vi "Write Context.vi"(8 "error in (no error)":errorcluster, 10 "context":string, 11 "URI in":refnum<class "URI.lvclass">) -> (0 "error out":errorcluster, 3 "URI out":refnum<class "URI.lvclass">)   [LabVIEW 2013, in "openURI.lvlib" / "URI.lvclass"]
uses:
  URI.lvclass
  URI.lvclass/URI.ctl
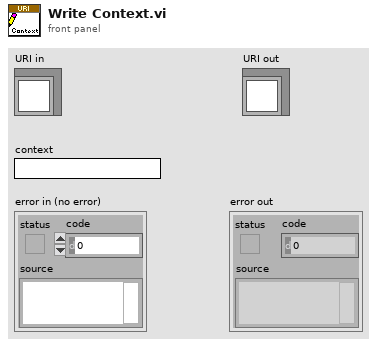
[diagram p1: front panel]
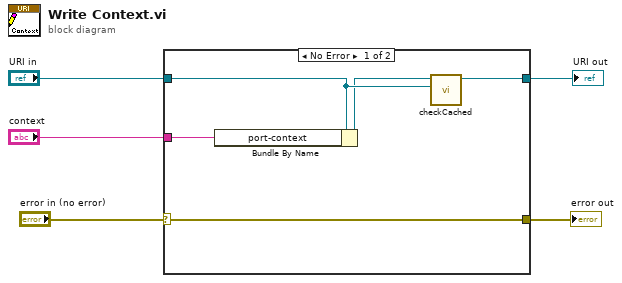
[diagram p0: block diagram]
diagram:
  n1 = case shown="No Error" "error in (no error)" {
    selector: "error in (no error)" -> [w9 w11]
    tunnel: "URI in" -> [w8 w12]
    tunnel: "context" -> [w10 _]
    tunnel: [w6 w12] -> w3
    tunnel: [w9 w11] -> w1
    frame No Error {
      n2 = Bundle By Name(cluster=w8, "port-context"=w10) -> (w7:refnum<class "URI.lvclass">)
      n3 = call "checkCached.vi"("Old"=w8, "New URI"=w7) -> ("URI"=w6:refnum<class "URI.lvclass">)  [unwired: 9 in]
    }
    frame Error {
    }
  }
  "URI out" <- w3
  "error out" <- w1
